vi "Constructor.vi"(5 "TimeZoneInfoId":string, 7 "OpenTime":timestamp, 8 "error in":errorcluster, 10 "DefectId":string, 11 "Name":string) -> (0 "error out":errorcluster, 3 "Defect":refnum<class "Defect.lvclass">)   [LabVIEW 2021, in "ProligentXMLGenerator.lvlib" / "Defect.lvclass"]
uses:
  Defect.lvclass
  Defect.lvclass/Defect.ctl
  Base/DateTime/DateTime.lvclass
  Model/UserComment/UserComment.lvclass
  Data.ctl
  Base/Guid/Guid.lvclass
  Model/CustomData/CustomData.lvclass
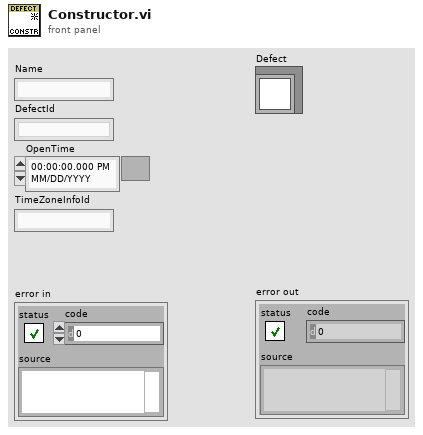
[diagram p1: front panel]
types:
  T1 = typedef "ProligentXMLGenerator.lvlib/Defect.lvclass/Data.ctl" = cluster{"Name":string, "Comments":refnum<class "UserComment.lvclass">[], "CustomData":refnum<class "CustomData.lvclass">, "DefectId":refnum<class "Guid.lvclass">, "OpenTime":refnum<class "DateTime.lvclass">, "TimeZoneInfoId":string}
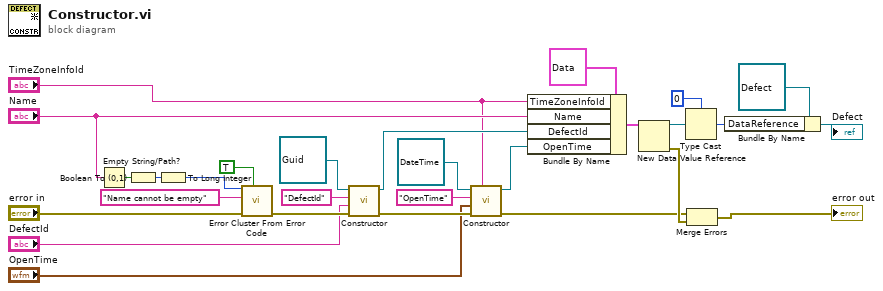
[diagram p0: block diagram]
diagram:
  n1 = Empty String/Path?(string/path="Name") -> (empty?=w14:bool)
  n2 = Boolean To (0,1)(Boolean=w14) -> (0, 1=w13:i16)
  n3 = To Long Integer(number=w13) -> (32bit integer=w12:i32)
  n4 = call <vilib>:"Error Cluster From Error Code.vi"("show call chain? (False)"=TRUE, "error in (no error)"="error in", "error message (\"\")"="Name cannot be empty" ("error message (\"\")"), "error code (0)"=w12) -> ("error out"=w7:errorcluster)  [unwired: 5 in]
  n5 = call-dynamic "Constructor.vi"("error in"=w7, "Value"="DefectId", "Name"="DefectId", "String in"=refnum<class "Guid.lvclass"> refnum ("ProligentCanonicalFile:Guid.lvclass")) -> ("error out"=w6:errorcluster, "String out"=w8:refnum<class "Guid.lvclass">)  [unwired: 6 in]
  n6 = call-dynamic "Constructor.vi"("TimeZoneInfoId"="TimeZoneInfoId", "error in"=w6, "Value"="OpenTime", "Name"="OpenTime", "DateTime in"=refnum<class "DateTime.lvclass"> refnum) -> ("error out"=w5:errorcluster, "DateTime out"=w17:refnum<class "DateTime.lvclass">)  [unwired: 5 in]
  n7 = Bundle By Name(cluster=T1 {"Name"="", "Comments"=[], "CustomData"=refnum, "DefectId"=refnum, "OpenTime"=refnum, "TimeZoneInfoId"=""} ("Data"), "TimeZoneInfoId"="TimeZoneInfoId", "Name"="Name", "DefectId"=w8, "OpenTime"=w17) -> (w22:T1)
  n8 = New Data Value Reference(data value=w22) -> (data value reference=w21:refnum<data-value>, error out=w18:errorcluster)  [unwired: 1 in]
  n9 = Type Cast(type=u64 0, x=w21) -> (*(type *) &x=w19:u64)
  n10 = Merge Errors(w5, w18) -> (→"error out":errorcluster)
  n11 = Bundle By Name(cluster=refnum<class "Defect.lvclass"> refnum ("ProligentResultProcessor:Defect"), "DataReference"=w19) -> (→"Defect":refnum<class "Defect.lvclass">)
